vi "Test3D.vi"() -> ()   [LabVIEW 2014]
uses:
  <vilib>/picture/3D Picture Control/Object/Create Object (name).vi
  <vilib>/picture/3D Picture Control/NI_3D Picture Control.lvlib
panel:
  in  "Alpha":sgl
  in  "Color Box":u32(colorbox)=16711680
  in  "STL Path":path
  out "3D Picture":refnum<vi>(3d-picture)
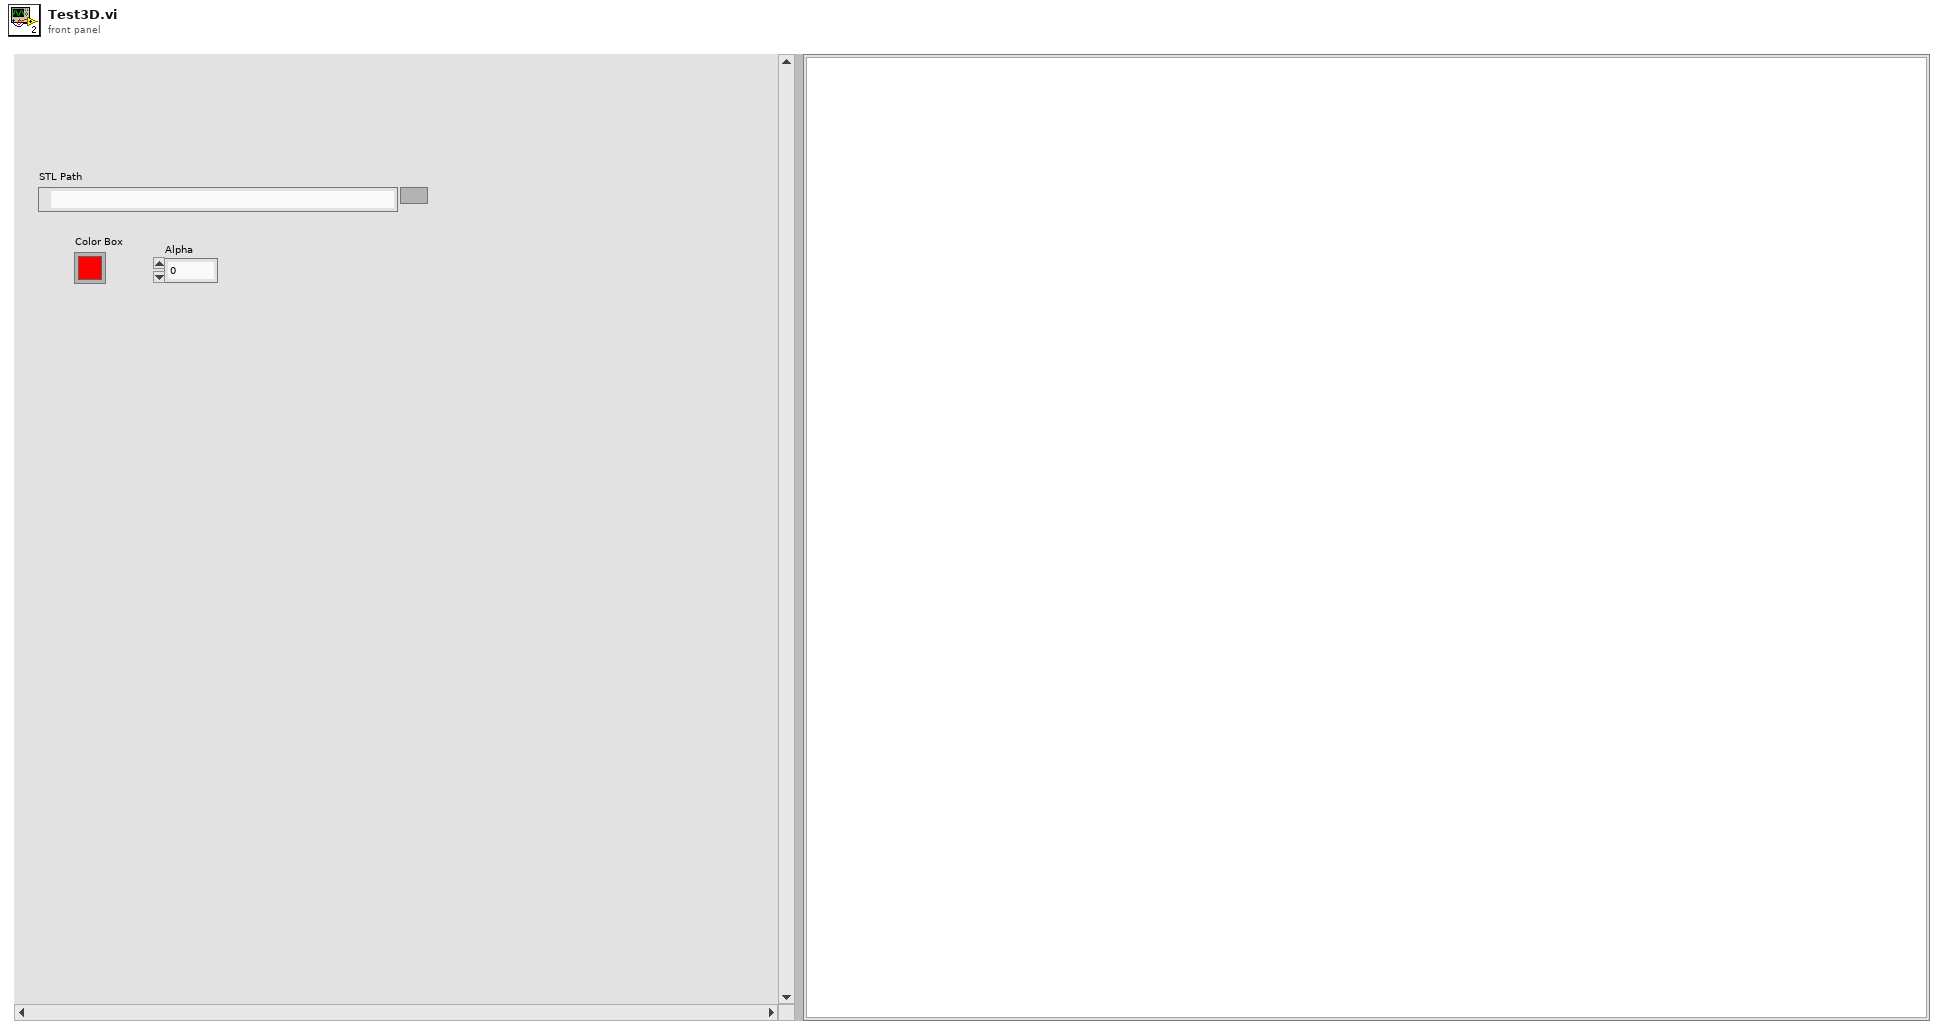
[diagram p1: front panel]
types:
  T1 = enum16{"Overall", "Per Primitive", "Per Vertex", "Binding Off"}
  T2 = enum16{"Points", "Lines", "Line Strip", "Line Loop", "Triangles", "Triangle Strip", "Triangle Fan", "Quads", "Quad Strip", "Polygon"}
  T3 = cluster{"Red":sgl, "Green":sgl, "Blue":sgl, "Alpha":sgl}
  T4 = typedef "TriangleFace.ctl" = cluster{"Normal":T5, "Vertex1":T5, "Vertex2":T5, "Vertex3":T5}
  T5 = typedef "Point3D.ctl" = cluster{"X":sgl, "Y":sgl, "Z":sgl}
  T6 = cluster{"Red":sgl, "Green":sgl, "Blue":sgl, "Alpha":sgl}[]
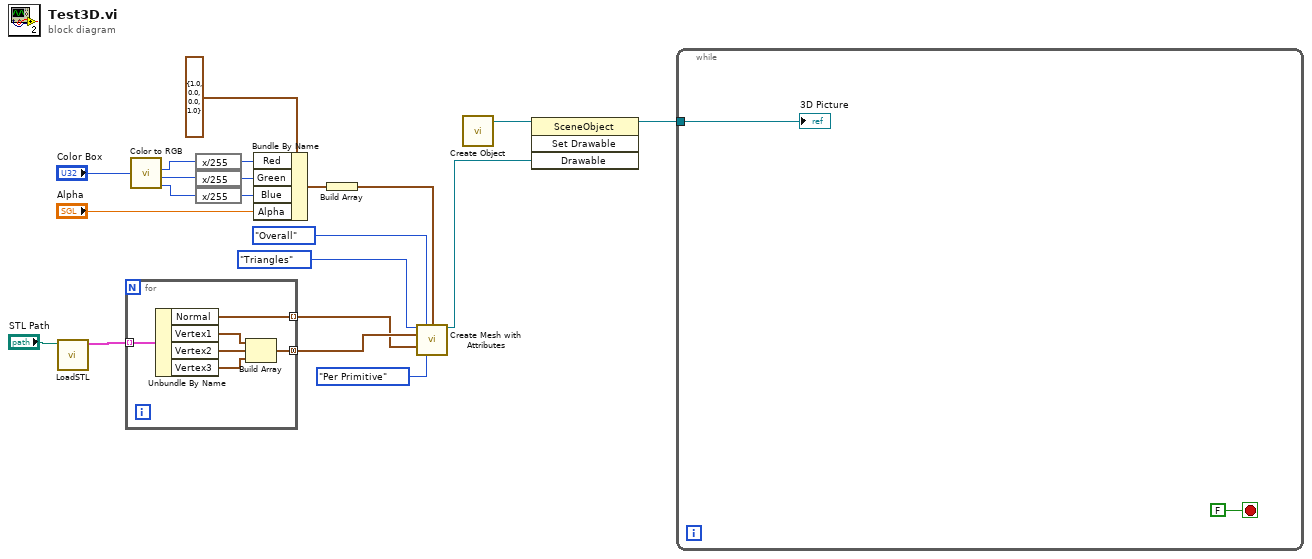
[diagram p0: block diagram]
diagram:
  n1 = call "LoadSTL.vi"("STL Path"="STL Path") -> ("Triangles"=w20:T4[])  [unwired: 8 in, 2 out]
  n2 = for {
    tunnel: w20 -> [w27] mode=indexing
    tunnel: [w23] -> w13 mode=concatenating
    tunnel: [w22] -> w12 mode=indexing
    n3 = Unbundle By Name(w27) -> ("Normal"=w22:T5, "Vertex1"=w26:T5, "Vertex2"=w25:T5, "Vertex3"=w24:T5)
    n4 = Build Array(w26, w25, w24) -> (w23:T5[])
  }
  n5 = call <vilib>:"Color to RGB.vi"("Color"="Color Box") -> ("R"=w3:u8, "G"=w2:u8, "B"=w1:u8)  [unwired: 1 out]
  n6 = expression code="x/255"(w3) -> (w6:u8)
  n7 = expression code="x/255"(w2) -> (w5:u8)
  n8 = expression code="x/255"(w1) -> (w4:u8)
  n9 = Bundle By Name(cluster=T3 {"Red"=1.0, "Green"=0.0, "Blue"=0.0, "Alpha"=1.0} ("Color"), "Red"=w6, "Green"=w5, "Blue"=w4, "Alpha"="Alpha") -> (w17:T3)
  n10 = Build Array(w17) -> (w16:T6)
  n11 = call <vilib>:"Create Mesh with Attributes.vi"("Draw Mode"=T2."Triangles", "Color Binding Mode"=T1."Overall", "Color Array"=w16, "Vertex Array"=w13, "Normal Array"=w12, "Normal Binding Mode"=T1."Per Primitive") -> ("New Mesh Refnum"=w8:refnum<vi>)  [unwired: 8 in, 1 out]
  n12 = call-poly <vilib>:"Create Object.vi"() -> ("Scene:New Object"=w10:refnum<vi>)  [unwired: 10 in, 1 out]
  n13 = invoke class="SceneObject" method="Set Drawable"(reference=w10, "Drawable"=w8) -> (reference out=w9:refnum<vi>)  [unwired: 2 in, 3 out]
  n14 = while {
    tunnel: w9 -> [w29]
    stop <- FALSE stop-if-true
    "3D Picture" <- w29
  }
